vi "setReadFIFO.vi"(10 "ReadFIFO":refnum<class "IReadFIFO.lvclass">, 11 "Modbus in":refnum<class "Modbus.lvclass">) -> (3 "Modbus out":refnum<class "Modbus.lvclass">)   [LabVIEW 2015, in "RTModbus.lvlib" / "Modbus.lvclass"]
uses:
  Modbus.lvclass
  Common_RT_FPGA/IReadFIFO/IReadFIFO.lvclass
  Modbus.lvclass/Modbus.ctl
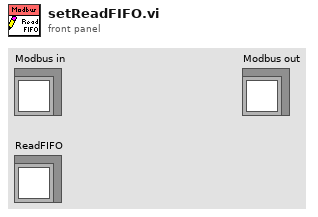
[diagram p1: front panel]
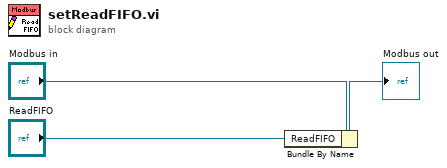
[diagram p0: block diagram]
diagram:
  n1 = Bundle By Name(cluster="Modbus in", "ReadFIFO"="ReadFIFO") -> (→"Modbus out":refnum<class "Modbus.lvclass">)
